vi "Unary helloworld_Greeter_SayHello.vi"(8 "error in":errorcluster, 10 "Request Data":T2, 11 "gRPC ID":T3) -> (0 "error out":errorcluster, 2 "Response Data":T1, 3 "gRPC ID out":T3)   [LabVIEW 2019, in "helloworld_client.lvlib"]
uses:
  helloworld_client.lvlib
  labview source/gRPC lv Support/grpc-lvsupport/grpcId.ctl
  RPC Messages/helloworld_HelloRequest.ctl
  RPC Messages/helloworld_HelloReply.ctl
  ca87ddad-a058-43bb-84a3-0da63f49ce15.vi
  labview source/gRPC lv Support/grpc-lvsupport/TranslateGrpcError.vi
  labview source/gRPC lv Support/grpc-lvsupport/Create Occurance.vi
  labview source/gRPC lv Support/grpc-lvsupport/Get Server Debug DLL Path.vi
  <vilib>/Utility/file.llb/Application Directory.vi
  <vilib>/Utility/error.llb/Error Cluster From Error Code.vi
  labview source/gRPC lv Support/grpc-lvsupport/Wait On Occurrence.vi
  labview source/gRPC lv Support/grpc-lvsupport/grpc-lvsupport.lvlib
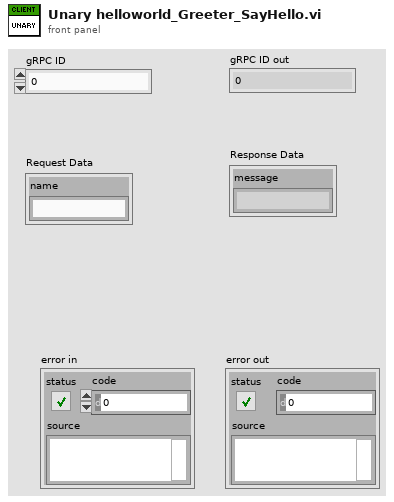
[diagram p1: front panel]
types:
  T1 = typedef "helloworld_client.lvlib/helloworld_HelloReply.ctl" = cluster{"message":string}
  T2 = typedef "helloworld_client.lvlib/helloworld_HelloRequest.ctl" = cluster{"name":string}
  T3 = typedef "grpc-lvsupport.lvlib/grpcId.ctl" = u64
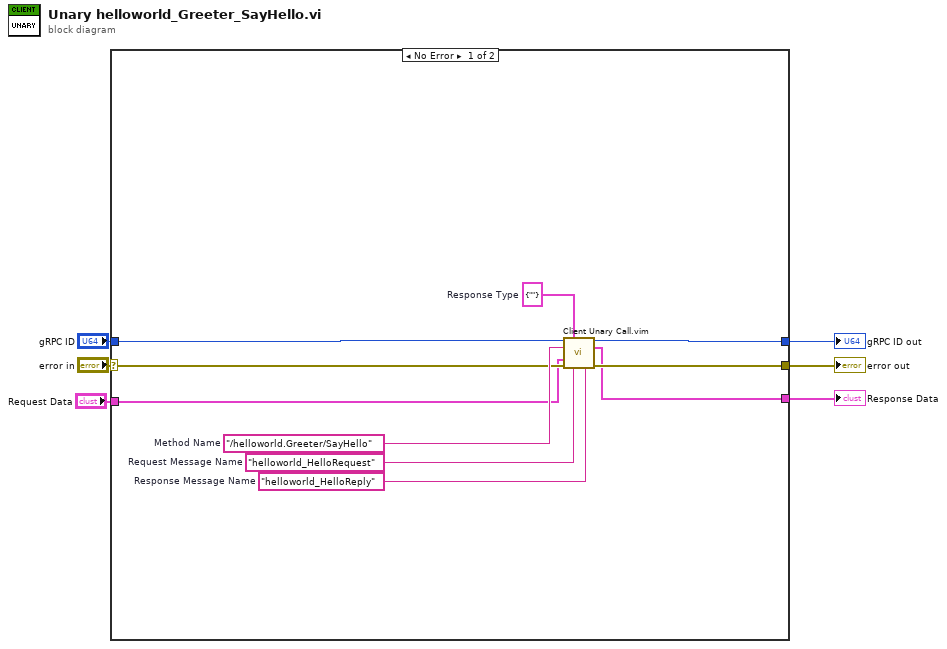
[diagram p0: block diagram]
diagram:
  n1 = case shown="No Error" "error in" {
    selector: "error in" -> [w12 w17]
    tunnel: [w11 w17] -> w5
    tunnel: "gRPC ID" -> [w10 w18]
    tunnel: [w9 w18] -> w3
    tunnel: "Request Data" -> [w8 _]
    tunnel: [w7 _] -> w1
    frame No Error {
      w13 = "helloworld_HelloReply"  # Response Message Name
      w14 = "helloworld_HelloRequest"  # Request Message Name
      w15 = T1 {"message"=""}  # Response Type
      w16 = "/helloworld.Greeter/SayHello"  # Method Name
      n2 = call "Client Unary Call.vim"("ClientID in"=w10, "Response Type"=w15, "Method Name"=w16, "Request Data"=w8, "error in"=w12, "Request Message Name"=w14, "Response Message Name"=w13) -> ("ClientID out"=w9:T3, "Response Data"=w7:T1, "error out"=w11:errorcluster)  [unwired: 6 in]
    }
    frame Error {
    }
  }
  "error out" <- w5
  "gRPC ID out" <- w3
  "Response Data" <- w1
